vi "error_missing_method.vi"(8 "error in (no error)":errorcluster, 11 "plugin":refnum<class "lv-post-installer.lvclass">) -> (0 "error out":errorcluster)   [LabVIEW 2015, in "lv-post-installer.lvlib"]
uses:
  lv-post-installer.lvlib
  classes/lv-post-installer/lv-post-installer.lvclass
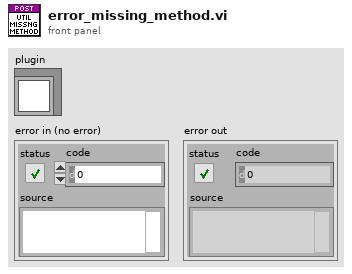
[diagram p1: front panel]
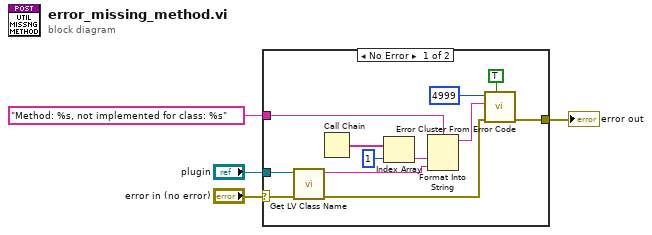
[diagram p0: block diagram]
diagram:
  n1 = case shown="No Error" "error in (no error)" {
    selector: "error in (no error)" -> [w9 w17]
    tunnel: "Method: %s, not implemented for class: %s" ("format string") -> [w15 _]
    tunnel: "plugin" -> [w12 _]
    tunnel: [w5 w17] -> w2
    frame No Error {
      n2 = call <vilib>:"Get LV Class Name.vi"("error in (no error)"=w9, "object"=w12) -> ("error out"=w8:errorcluster, "class name"=w11:string)  [unwired: 8 in]
      n3 = Call Chain() -> (call chain=w14:string[])
      n4 = Index Array(array=w14, index=1) -> (element=w10:string)
      n5 = Format Into String(format string=w15, w10, w11) -> (resulting string=w7:string)  [unwired: 2 in, 1 out]
      n6 = call <vilib>:"Error Cluster From Error Code.vi"("show call chain? (False)"=TRUE, "error in (no error)"=w8, "error message (\"\")"=w7, "error code (0)"=4999) -> ("error out"=w5:errorcluster)  [unwired: 5 in]
    }
    frame Error {
    }
  }
  "error out" <- w2
